vi "Read Homing Parameters.vi"(8 "error in (no error)":errorcluster, 11 "Filter Wheel in":refnum<class "Filter Wheel.lvclass">) -> (0 "error out":errorcluster, 2 "Homing Parameters":T1, 3 "Filter Wheel out":refnum<class "Filter Wheel.lvclass">)   [LabVIEW 2022 SP3, in "Filter Wheel.lvclass"]
uses:
  Filter Wheel.lvclass
  Filter Wheel Arduino Control/Filter Wheel Arduino Homing cluster.ctl
  Filter Wheel.lvclass/Filter Wheel.ctl
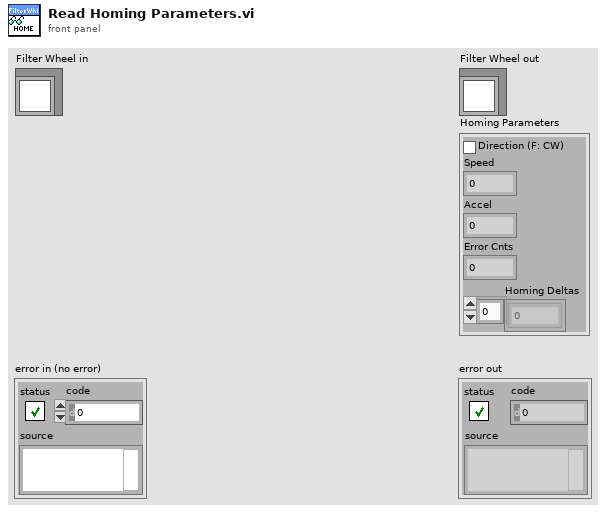
[diagram p1: front panel]
types:
  T1 = typedef "Filter Wheel Arduino Homing cluster.ctl" = cluster{"Direction (F: CW)":bool, "Speed":i32, "Accel":i32, "Error Cnts":i32, "Homing Deltas":i32[]}
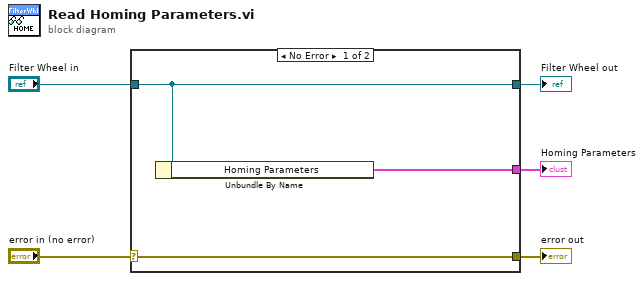
[diagram p0: block diagram]
diagram:
  n1 = case shown="No Error" "error in (no error)" {
    selector: "error in (no error)" -> [w8 w9]
    tunnel: [w8 w9] -> w4
    tunnel: [w7 w10] -> w2
    tunnel: "Filter Wheel in" -> [w7 w10]
    tunnel: [w6 _] -> w1
    frame No Error {
      n2 = Unbundle By Name(w7) -> ("Homing Parameters"=w6:T1)
    }
    frame Error {
    }
  }
  "error out" <- w4
  "Filter Wheel out" <- w2
  "Homing Parameters" <- w1
